vi "String.vi"(7 "data type of variable":string, 8 "error in":errorcluster, 10 "variable name":string, 11 "pipe in":T1) -> (0 "error out":errorcluster, 2 "value":string, 3 "pipe out":T1)   [LabVIEW 2013, in "GOLPI library.lvlib"]
uses:
  GOLPI library.lvlib
  LV Process.lvlibp/Pipe Handle.ctl
  Globals.vi
  <vilib>/Utility/error.llb/Error Cluster From Error Code.vi
  <vilib>/regexp/Match Regular Expression.xnode
  <vilib>/ErrorRing/Error Ring.xnode
  LV Process.lvlibp
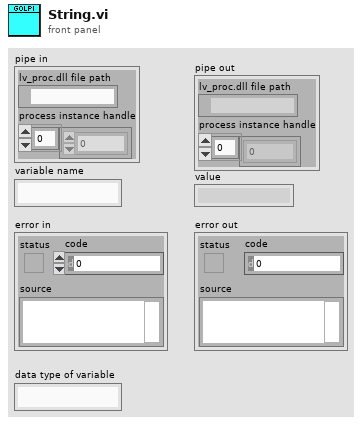
[diagram p1: front panel]
types:
  T1 = typedef "LV Process.lvlibp/Pipe Handle.ctl" = cluster{"lv_proc.dll file path":path, "process instance handle":u32[]}
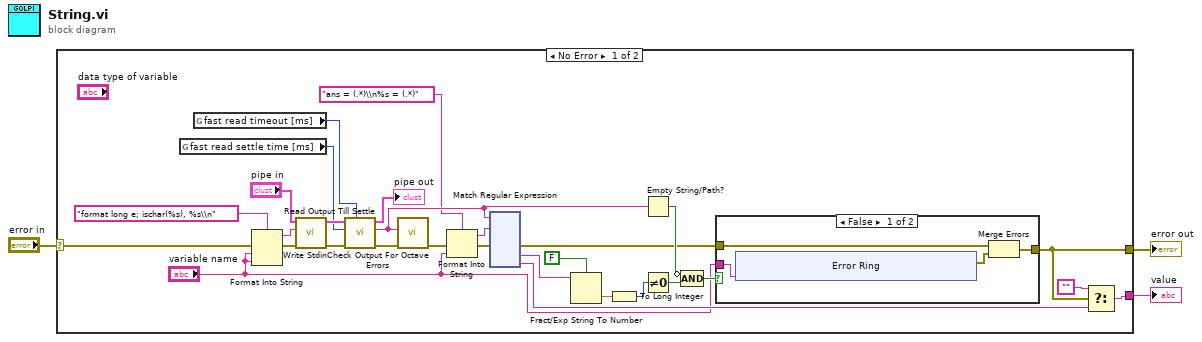
[diagram p0: block diagram]
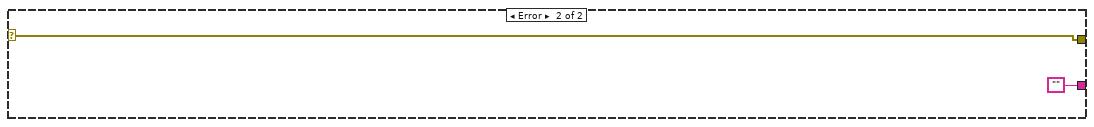
[diagram p3: hidden frame]
diagram:
  n1 = case shown="No Error" "error in" {
    selector: "error in" -> [w9 w162]
    tunnel: [w20 w162] -> w3
    tunnel: [w19 ""] -> w2
    frame No Error {
      n2 = global read "Globals.vi" "fast read settle time [ms]"() -> (w15:u32)
      n3 = global read "Globals.vi" "fast read timeout [ms]"() -> (w14:u32)
      n4 = Format Into String(format string="format long e; ischar(%s), %s\\n", error in=w9, "variable name", "variable name") -> (resulting string=w22:string, error out=w10:errorcluster)  [unwired: 1 in]
      n5 = call "Write Stdin.vi"("error in"=w10, "write buffer"=w22, "pipe in"="pipe in") -> ("error out"=w16:errorcluster, "pipe out"=w31:T1)  [unwired: 6 in, 1 out]
      n6 = call "Read Output Till Settle.vi"("timeout [ms]"=w14, "error in"=w16, "settled for [ms]"=w15, "pipe in"=w31) -> ("error out"=w21:errorcluster, "read buffer"=w13:string, "pipe out"=→"pipe out":T1)  [unwired: 4 in, 1 out]
      n7 = call "Check Output For Octave Errors.vi"("error in"=w21, "read buffer"=w13) -> ("error out"=w6:errorcluster)  [unwired: 9 in]
      n8 = Format Into String(format string="ans = (.*)\\n%s = (.*)" ("regular expression"), error in=w6, "variable name") -> (resulting string=w7:string, error out=w5:errorcluster)  [unwired: 1 in]
      n9 = xnode "Match Regular Expression"("input string"=w13, "regular expression"=w7, "error in"=w5) -> ("error out"=w12:errorcluster, "submatch 1"=w29:string, "submatch 2"=w17:string)  [unwired: 3 in, 4 out]
      n10 = Fract/Exp String To Number(use system decimal point (T)=FALSE, string=w29) -> (number=w28:dbl)  [unwired: 2 in, 1 out]
      n11 = To Long Integer(number=w28) -> (32bit integer=w27:i32)
      n12 = Empty String/Path?(string/path=w13) -> (empty?=w25:bool)
      n13 = Not Equal To 0?(x=w27) -> (x != 0?=w26:bool)
      n14 = Compound Arithmetic op=AND(invert w25, w26) -> (w24:bool)
      n15 = case shown="False" w24 {
        tunnel: [w34 w44] -> w20
        tunnel: w12 -> [w35 w44]
        tunnel: "variable name" -> [w33 _]
        frame False {
          n16 = xnode "Error Ring"("parameter 0"=w33) -> ("error out"=w36:errorcluster)
          n17 = Merge Errors(w35, w36) -> (w34:errorcluster)
        }
        frame True {
        }
      }
      n18 = Select(t="", s=w20, f=w17) -> (s? t:f=w19:string)
    }
    frame Error {
    }
  }
  "value" <- w2
  "error out" <- w3
